vi "Test Generated Voltage Ramp Duration Correct.vi"(8 "error in (no error)":errorcluster, 11 "Ramp Voltage Test In":refnum<class "Ramp Voltage Test.lvclass">) -> (0 "error out":errorcluster, 3 "Ramp Voltage Test Out":refnum<class "Ramp Voltage Test.lvclass">)   [LabVIEW 2020, in "High Level PSU With Tests.lvlib" / "Ramp Voltage Test.lvclass"]
uses:
  Ramp Voltage Test.lvclass
  C:/Program Files (x86)/National Instruments/LabVIEW 2020/vi.lib/Astemes/LUnit/Test Case.lvclass
  Ramp Voltage/Ramp Settings.ctl
  Ramp Voltage/Ramp Voltage.lvclass
  <vilib>/Astemes/LUnit/Test Case.lvclass/Test Case.ctl
  01074fa8-ee8a-411d-bc8b-fc92c4f90959.vi
  <vilib>/Astemes/LUnit/Palette/Pass.vi
  <vilib>/Astemes/LUnit/Palette/Fail.vi
  <vilib>/Astemes/LUnit/Compare Variants.vi
  <vilib>/Astemes/LUnit/Describe Comparison.vi
  <vilib>/Astemes/LUnit/Set Assertion Type.vi
  <vilib>/Astemes/LUnit/Add test result.vi
  <vilib>/Astemes/LUnit/Variant to string.vi
  <vilib>/Astemes/LUnit/LUnit Record Assertion Result.vi
  <vilib>/Astemes/LUnit/LUnit Aggregate Assertion Results.vi
  <vilib>/Astemes/LUnit/Method Result/LUnit Merge Status.vi
  <vilib>/Astemes/LUnit/LUnit Concatenate result strings.vi
  <vilib>/Utility/Data Type/Get Type Information.vi
  <vilib>/Utility/LVClass/Get LV Class Name.vi
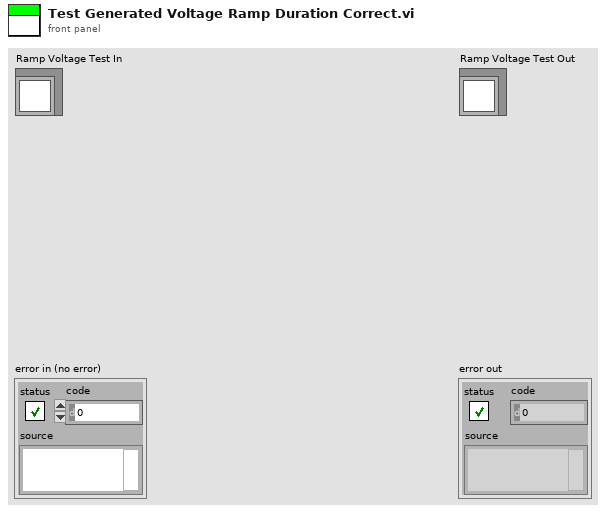
[diagram p1: front panel]
types:
  T1 = typedef "High Level PSU With Tests.lvlib/Ramp Voltage.lvclass/Ramp Settings.ctl" = cluster{"Max Output Voltage [V]":dbl, "Min Output Voltage [V]":dbl, "Step Size [V]":dbl, "Ramp Time [s]":dbl}
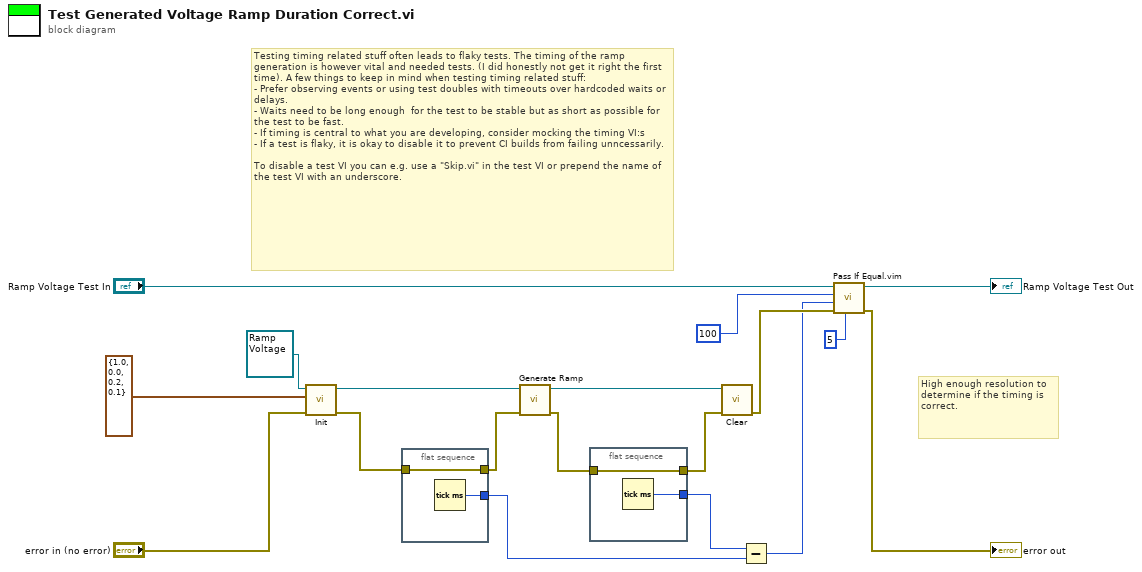
[diagram p0: block diagram]
diagram:
  # "High enough resolution to determine if the timing is correct."
  # "Testing timing related stuff often leads to flaky tests. The timing of the ramp generation is however vital and needed tests. (I did honestly not get it right the first time). A few things to keep in mind when testing timing related stuff:\n- Prefer observing events or using test doubles with timeouts over hardcoded waits or delays.\n- Waits need to be long enough  for the test to be stable but as short as possible for the test to be fast.\n- If timing is central to what you are developing, consider mocking the timing VI:s\n- If a test is flaky, it is okay to disable it to prevent CI builds from failing unncessarily. \n\nTo disable a test VI you can e.g. use a \"Skip.vi\" in the test VI or prepend the name of the test VI with an underscore."
  n1 = call "Init.vi"("error in (no error)"="error in (no error)", "Settings"=T1 {"Max Output Voltage [V]"=1.0, "Min Output Voltage [V]"=0.0, "Step Size [V]"=0.2, "Ramp Time [s]"=0.1}, "Ramp Voltage In"=refnum<class "Ramp Voltage.lvclass"> refnum ("Ramp Use Case In")) -> ("error out"=w9:errorcluster, "Ramp Voltage Out"=w15:refnum<class "Ramp Voltage.lvclass">)  [unwired: 7 in]
  n2 = flat-sequence {
    tunnel: w9 -> [w20]
    tunnel: [w20] -> w8
    tunnel: [w19] -> w4
    frame #0 {
      n3 = Tick Count (ms)() -> (millisecond timer value=w19:u32)
    }
  }
  n4 = call "Generate Ramp.vi"("error in (no error)"=w8, "Ramp Use Case In"=w15) -> ("error out"=w6:errorcluster, "Ramp Use Case Out"=w11:refnum<class "Ramp Voltage.lvclass">)  [unwired: 8 in]
  n5 = flat-sequence {
    tunnel: [w22] -> w7
    tunnel: w6 -> [w22]
    tunnel: [w21] -> w5
    frame #0 {
      n6 = Tick Count (ms)() -> (millisecond timer value=w21:u32)
    }
  }
  n7 = call "Clear.vi"("error in (no error)"=w7, "Ramp Use Case in"=w11) -> ("error out"=w12:errorcluster)  [unwired: 8 in, 1 out]
  n8 = Subtract(x=w5, y=w4) -> (x-y=w3:u32)
  n9 = call "Pass If Equal.vim"("Delta"=u32 5 ("x-y"), "error in (no error)"=w12, "Actual"=w3, "Expected"=u32 100 ("x-y"), "LUnit Test Case In"="Ramp Voltage Test In") -> ("error out"=→"error out":errorcluster, "LUnit Test Case Out"=→"Ramp Voltage Test Out":refnum<class "Ramp Voltage Test.lvclass">)  [unwired: 5 in]
